vi "EDDSequenceBulilder.vi"(8 "Due Dates":u16[](array[numeric]), 9 "Number Of Machines":i32=8, 10 "Number Of Operations":i32=64, 11 "Proocessing Times MxJ":u16[][](array[numeric])) -> (2 "EDD Squence":i32[](array[numeric]), 3 "Flattened Processing Times":u16[](array[numeric]))   [LabVIEW 2013]
panel:
  out "Due Date Sorted Job Order":i32[](array[numeric])
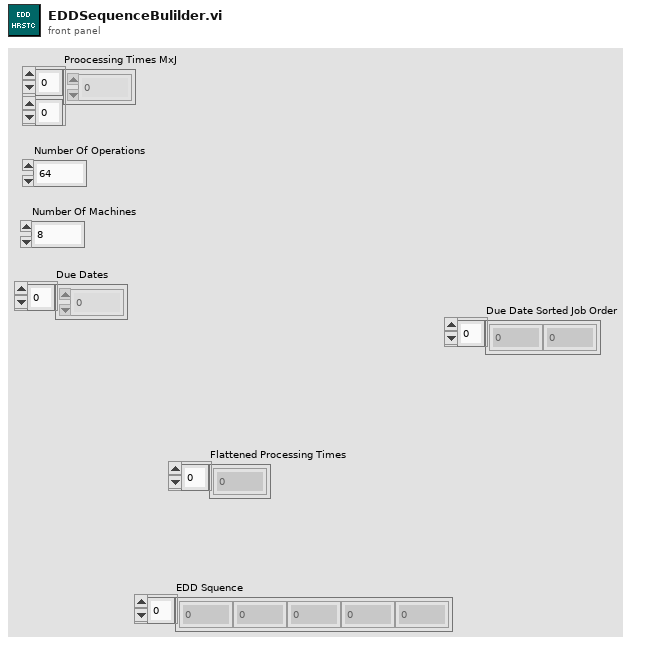
[diagram p1: front panel]
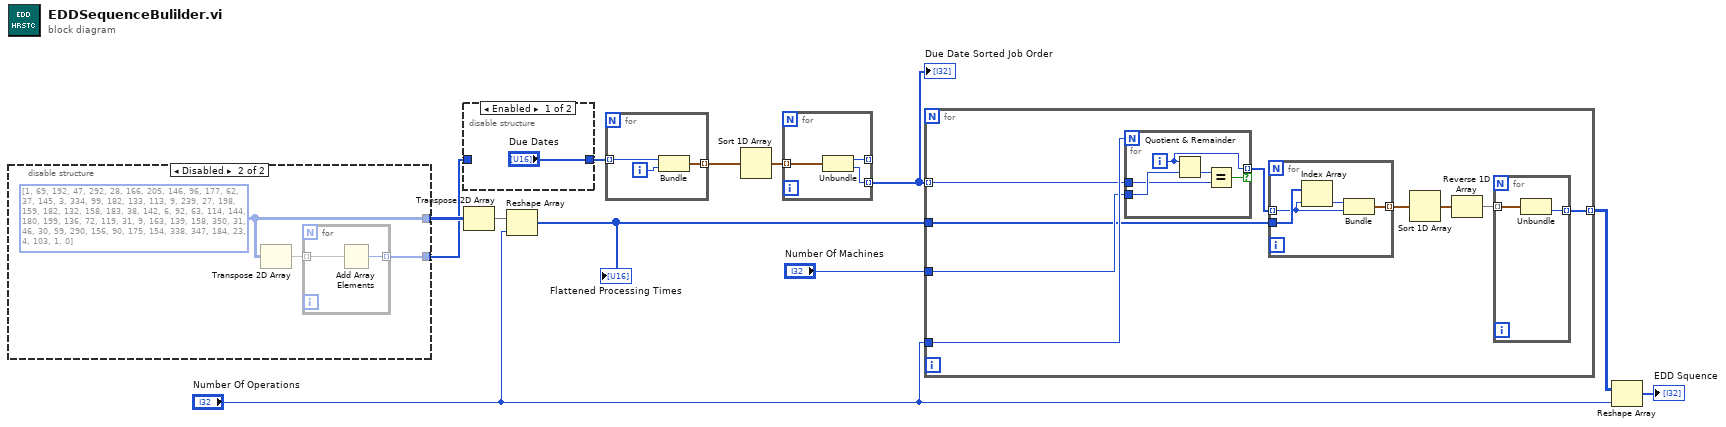
[diagram p0: block diagram]
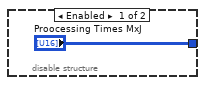
[diagram p3: hidden frame]
diagram:
  n1 = disable-structure shown="Disabled" {
    disable-tunnel: ["Proocessing Times MxJ" w16] -> w12
    disable-tunnel: [_ w15] -> w5
    frame Enabled {
    }
    frame Disabled {
      w16 = u16[][] [[1, 69, 192, 47, 292, 28, 166, 205], [146, 96, 177, 62, 37, 145, 3, 334], [99, 182, 133, 113, 9, 239, 27, 198], [159, 182, 132, 158, 183, 38, 142, 6], [92, 63, 114, 144, 180, 199, 136, 72], [119, 31, 9, 163, 139, 158, 350, 31], [46, 30, 59, 290, 156, 90, 175, 154], [338, 347, 184, 23, 4, 103, 1, 0]] ("Proocessing Times (8x8)")
      n2 = Transpose 2D Array(2D array=w16) -> (transposed array=w14:u16[][])
      n3 = for {
        tunnel: w14 -> [w18] mode=indexing
        tunnel: [w17] -> w15 mode=indexing
        n4 = Add Array Elements(numeric array=w18) -> (sum=w17:u16)
      }
    }
  }
  n5 = disable-structure shown="Enabled" {
    disable-tunnel: ["Due Dates" w20] -> w10
    disable-tunnel: w5 -> [_ w20]
    frame Enabled {
    }
    frame Disabled {
    }
  }
  n6 = Transpose 2D Array(2D array=w12) -> (transposed array=w11:u16[][])
  n7 = Reshape Array(w11, "Number Of Operations") -> (w4:u16[])
  "Flattened Processing Times" <- w4
  n8 = for {
    tunnel: w10 -> [w23] mode=indexing
    tunnel: [w21] -> w9 mode=indexing
    i -> [w22]
    n9 = Bundle(w23, w22) -> (w21:cluster{u16, i32})  [unwired: 1 in]
  }
  n10 = Sort 1D Array(array=w9) -> (sorted array=w8:cluster{u16, i32}[])
  n11 = for {
    tunnel: w8 -> [w26] mode=indexing
    tunnel: [w25] -> _ mode=indexing
    tunnel: [w24] -> w7 mode=indexing
    n12 = Unbundle(w26) -> (w25:u16, w24:i32)
  }
  "Due Date Sorted Job Order" <- w7
  n13 = for {
    tunnel: "Number Of Operations" -> [w35]
    tunnel: w7 -> [w34] mode=indexing
    tunnel: "Number Of Machines" -> [w33]
    tunnel: [w27] -> w3 mode=indexing
    tunnel: w4 -> [w31]
    n14 = for {
      N: w35 -> [_]
      tunnel: w34 -> [w44]
      tunnel: w33 -> [w46]
      tunnel: [w43] -> w32 mode=indexing if=w42
      i -> [w43]
      n15 = Quotient & Remainder(x=w43, y=w46) -> (floor(x/y)=w45:i32)  [unwired: 1 out]
      n16 = Equal?(x=w45, y=w44) -> (x = y?=w42:bool)
    }
    n17 = for {
      tunnel: w32 -> [w39] mode=indexing
      tunnel: w31 -> [w41]
      tunnel: [w38] -> w30 mode=indexing
      n18 = Index Array(array=w41, index=w39) -> (element=w40:u16)
      n19 = Bundle(w40, w39) -> (w38:cluster{u16, i32})  [unwired: 1 in]
    }
    n20 = Sort 1D Array(array=w30) -> (sorted array=w29:cluster{u16, i32}[])
    n21 = Reverse 1D Array(array=w29) -> (reversed array=w28:cluster{u16, i32}[])
    n22 = for {
      tunnel: w28 -> [w37] mode=indexing
      tunnel: [w36] -> w27 mode=indexing
      n23 = Unbundle(w37) -> (w36:i32)  [unwired: 1 out]
    }
  }
  n24 = Reshape Array(w3, "Number Of Operations") -> (→"EDD Squence":i32[])
